vi "Get Instr Ident.vi"(8 "error in":errorcluster, 11 "CFG JSON in":refnum<class "CFG JSON.lvclass">) -> (0 "error out":errorcluster, 2 "Instr Ident":string, 3 "CFG JSON out":refnum<class "CFG JSON.lvclass">)   [LabVIEW 2024, in "HAL.lvlib" / "CFG JSON.lvclass"]
uses:
  CFG JSON.lvclass
  2eafeabf-da49-4e57-aee5-502056b959b8.vi
  2eafeabf-da49-4e57-aee5-502056b959b8.vi/a4169a97-72fc-4003-a778-603cf20cafa0.vi
  <vilib>/JDP Science/JSONtext/Find Item.vi
  <vilib>/JDP Science/JSONtext/Next JSON Value.vi
  <vilib>/JDP Science/JSONtext/String Subset.vi
  <vilib>/JDP Science/JSONtext/Parsing/Advance past next JSON Value (inlined COPY).vi
  <vilib>/JDP Science/JSONtext/Parsing/Advance past whitespace.vi
  <vilib>/JDP Science/JSONtext/Parsing/Advance past String.vi
  <vilib>/JDP Science/JSONtext/Parsing/Advance past Number.vi
  <vilib>/JDP Science/JSONtext/Parsing/Advance past Line Ending.vi
  <vilib>/JDP Science/JSONtext/Parsing/Parse Full Path or Item Name.vi
  <vilib>/JDP Science/JSONtext/Parsing/Advance past Array.vi
  <vilib>/JDP Science/JSONtext/Parsing/Advance past Object.vi
  <vilib>/JDP Science/JSONtext/support/Error Cluster From Code.vi
  <vilib>/JDP Science/JSONtext/Offset/Find Item Locations by Path.vi
  <vilib>/JDP Science/JSONtext/JSON text to Variant.vi
  <vilib>/Utility/error.llb/Error Cluster From Error Code.vi
  CFG Base/CFG Base.lvclass
  <vilib>/JDP Science/JSONtext/LVClass Serializer/JSONtext LVClass Serializer.lvclass
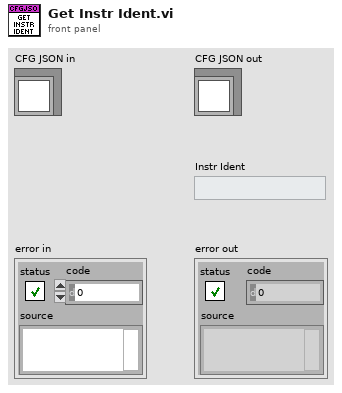
[diagram p1: front panel]
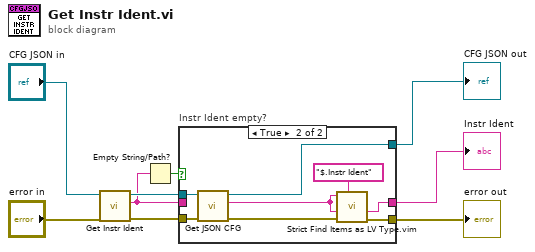
[diagram p0: block diagram]
diagram:
  n1 = call-parent "Get Instr Ident.vi"("error in"="error in", "CFG Base in"="CFG JSON in") -> ("error out"=w3:errorcluster, "Instr Ident"=w1:string, "CFG Base out"=w4:refnum<class "CFG JSON.lvclass">)  [unwired: 7 in]
  n2 = Empty String/Path?(string/path=w1) -> (empty?=w2:bool)
  n3 = case "Instr Ident empty?" shown="True" w2 {
    tunnel: [w10 w19] -> w9
    tunnel: [w11 w18] -> w8
    tunnel: [w12 w16] -> w7
    tunnel: w4 -> [w11 w14]
    tunnel: w3 -> [w10 w13]
    tunnel: w1 -> [w12 _]
    frame False {
    }
    frame True {
      n4 = call "Get JSON CFG.vi"("CFG JSON in"=w14) -> ("<JSON> CFG"=w17:string, "CFG JSON out"=w18:refnum<class "CFG JSON.lvclass">)  [unwired: 9 in]
      n5 = call "Strict Find Items as LV Type.vim"("$Path or Item Name"="$.Instr Ident", "error in"=w13, "Data Type and Default Value"=w17, "<JSON>"=w17) -> ("error out"=w19:errorcluster, "Data out"=w16:string)  [unwired: 5 in, 1 out]
    }
  }
  "error out" <- w9
  "CFG JSON out" <- w8
  "Instr Ident" <- w7
